vi "PutGetTreeNode Example.vi"() -> ()   [LabVIEW 2010]
uses:
  <vilib>/builds/MDSplus/MDSplus/MDSplus.lvlib
panel:
  in  "Path":string=":NUM0"
  in  "Tree Shot":i32=-1
  in  "Tree Name":string="my_tree"
  in  "Value In":sgl=5.555
  out "Value Out":sgl
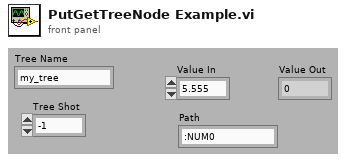
[diagram p1: front panel]
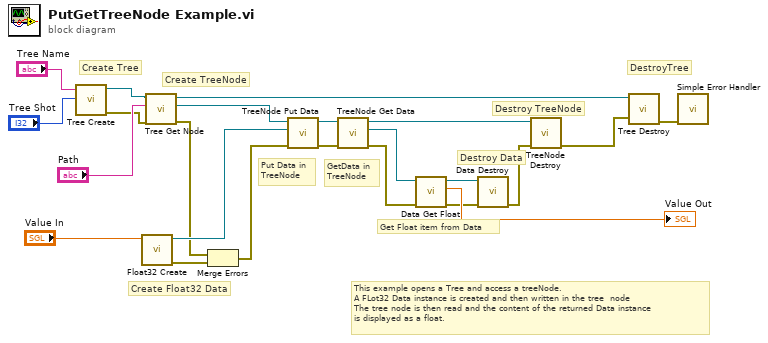
[diagram p0: block diagram]
diagram:
  # "This example opens a Tree and access a treeNode.\nA FLot32 Data instance is created and then written in the tree  node\nThe tree node is then read and the content of the returned Data instance\nis displayed as a float."
  # "DestroyTree"
  # "Destroy TreeNode"
  # "Destroy Data"
  # "Get Float item from Data"
  # "GetData in\nTreeNode"
  # "Put Data in\nTreeNode"
  # "Create Float32 Data"
  # "Create TreeNode"
  # "Create Tree"
  n1 = call <vilib>:"Tree Create.vi"("Shot"="Tree Shot", "Name"="Tree Name") -> ("error out"=w4:errorcluster, "Tree DVR out"=w3:refnum<data-value>)  [unwired: 8 in]
  n2 = call <vilib>:"Float32 Create.vi"("SGL in"="Value In") -> ("error out"=w19:errorcluster, "Float32 DVR out"=w21:refnum<data-value>)  [unwired: 9 in]
  n3 = call <vilib>:"Tree Get Node.vi"("error in (no error)"=w4, "Path"="Path", "Tree DVR in"=w3) -> ("error out"=w8:errorcluster, "Node out"=w9:refnum<data-value>, "Tree DVR out"=w2:refnum<data-value>)  [unwired: 6 in]
  n4 = Merge Errors(w8, w19) -> (w20:errorcluster)
  n5 = call <vilib>:"TreeNode Put Data.vi"("error in (no error)"=w20, "Data"=w21, "TreeNode DVR in"=w9) -> ("error out"=w17:errorcluster, "TreeNode DVR out"=w18:refnum<data-value>)  [unwired: 7 in]
  n6 = call <vilib>:"TreeNode Get Data.vi"("error in (no error)"=w17, "TreeNode DVR in"=w18) -> ("error out"=w15:errorcluster, "Data out"=w16:refnum<data-value>, "TreeNode DVR out"=w1:refnum<data-value>)  [unwired: 7 in]
  n7 = call <vilib>:"Data Get Float.vi"("error in (no error)"=w15, "Data DVR in"=w16) -> ("error out"=w12:errorcluster, "SGL out"=→"Value Out":sgl, "Data DVR out"=w14:refnum<data-value>)  [unwired: 7 in]
  n8 = call <vilib>:"Data Destroy.vi"("error in (no error)"=w12, "Data DVR in"=w14) -> ("error out"=w11:errorcluster)  [unwired: 9 in]
  n9 = call <vilib>:"TreeNode Destroy.vi"("error in (no error)"=w11, "TreeNode DVR in"=w1) -> ("error out"=w7:errorcluster)  [unwired: 9 in]
  n10 = call <vilib>:"Tree Destroy.vi"("error in (no error)"=w7, "Tree DVR in"=w2) -> ("error out"=w10:errorcluster)  [unwired: 9 in]
  n11 = call <vilib>:"Simple Error Handler.vi"("error in (no error)"=w10) -> ()  [unwired: 4 in, 5 out]
